vi "MakeBeverage.vi"(8 "Error In":errorcluster, 10 "Type":T1, 11 "reference in":refnum<class "BeverageFlyweightFactory.lvclass">) -> (0 "Error Out":errorcluster, 2 "Return(LabVIEW Class)":refnum<class "IBeverage.lvclass">, 3 "reference out":refnum<class "BeverageFlyweightFactory.lvclass">)   [LabVIEW 2020, in "BeverageFlyweightFactory.lvclass"]
uses:
  BeverageFlyweightFactory.lvclass
  BeverageType.ctl
  IBeverage_interface/IBeverage.lvclass
  BubbleMilkTea_class/BubbleMilkTea.lvclass
  C:/Projects/DesignPatterns/FlyweightPattern2/IBeverage_interface/IBeverage.lvclass
  FoamMilkTea_class/FoamMilkTea.lvclass
  OolingMilkTea_class/OolingMilkTea.lvclass
  CoconutMilkTea_class/CoconutMilkTea.lvclass
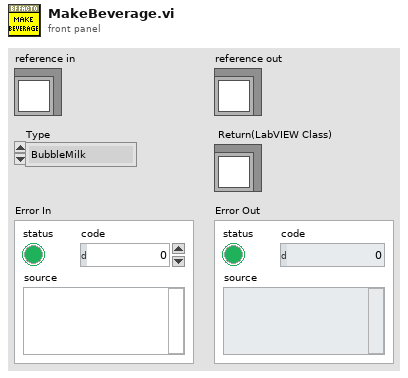
[diagram p1: front panel]
types:
  T1 = typedef "BeverageType.ctl" = enum16{"BubbleMilk", "FoamMilk", "OolongMilk", "CoconutMilk"}
  T2 = typedef "BeverageFlyweightFactory.lvclass/ObjectAttributes.ctl" = cluster{"_beverages":map{T1, refnum<class "IBeverage.lvclass">}}
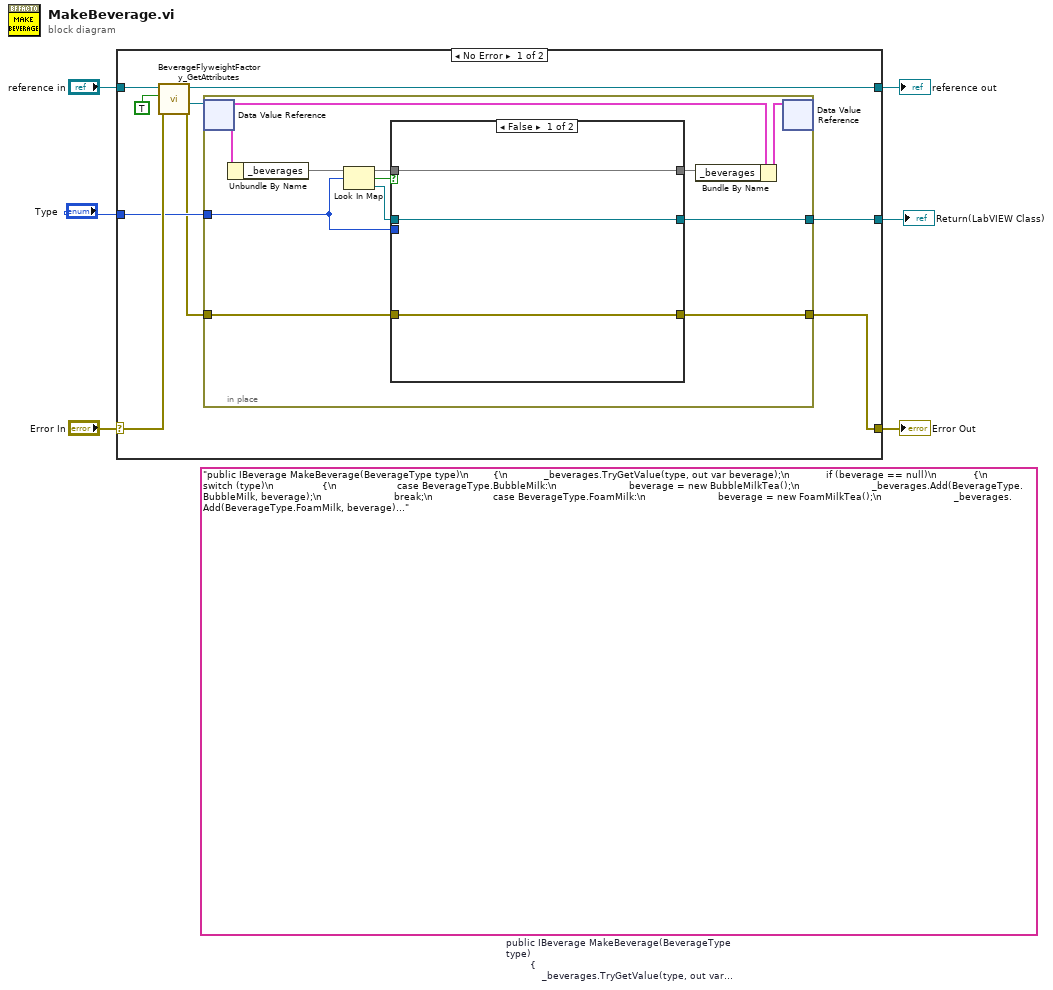
[diagram p0: block diagram]
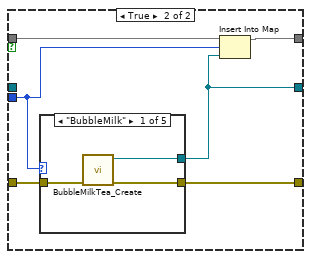
[diagram p2: hidden frame]
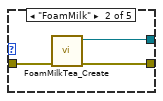
[diagram p3: hidden frame]
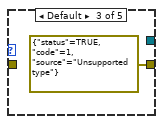
[diagram p4: hidden frame]
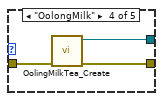
[diagram p5: hidden frame]
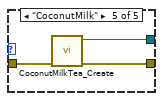
[diagram p6: hidden frame]
diagram:
  (unwired) "public IBeverage MakeBeverage(BeverageType type)\n        {\n            _beverages.TryGetValue(type, out var beverage);\n            if (beverage == null)\n            {\n                switch (type)\n                {\n                    case BeverageType.BubbleMilk:\n                        beverage = new BubbleMilkTea();\n                        _beverages.Add(BeverageType.BubbleMilk, beverage);\n                        break;\n                    case BeverageType.FoamMilk:\n                        beverage = new FoamMilkTea();\n                        _beverages.Add(BeverageType.FoamMilk, beverage);\n                        break;\n                    case BeverageType.OolongMilk:\n                        beverage = new OolingMilkTea();\n                        _beverages.Add(BeverageType.OolongMilk, beverage);\n                        break;\n                    case BeverageType.CoconutMilk:\n                        beverage = new CoconutMilkTea();\n                        _beverages.Add(BeverageType.CoconutMilk, beverage);\n                        break;\n                    default:\n                        throw new ArgumentOutOfRangeException(nameof(type), type, null);\n                }\n            }\n\n            return beverage;\n        }"  # public IBeverage MakeBeverage(BeverageType type)         {             _beverages.TryGetValue(type, out var beverage);             if (beverage == null)             {                 switch (type)                 {                     case BeverageType.BubbleMilk:                         beverage = new BubbleMilkTea();                         _beverages.Add(BeverageType.BubbleMilk, beverage);                         break;                     case BeverageType.FoamMilk:                         beverage = new FoamMilkTea();                         _beverages.Add(BeverageType.FoamMilk, beverage);                         break;                     case BeverageType.OolongMilk:                         beverage = new OolingMilkTea();                         _beverages.Add(BeverageType.OolongMilk, beverage);                         break;                     case BeverageType.CoconutMilk:                         beverage = new CoconutMilkTea();                         _beverages.Add(BeverageType.CoconutMilk, beverage);                         break;                     default:                         throw new ArgumentOutOfRangeException(nameof(type), type, null);                 }             }              return beverage;         }
  n1 = case shown="No Error" "Error In" {
    selector: "Error In" -> [w14 w49]
    tunnel: [w7 w49] -> w5
    tunnel: [w13 w48] -> w3
    tunnel: "reference in" -> [w15 w48]
    tunnel: "Type" -> [w10 _]
    tunnel: [w9 _] -> w1
    frame No Error {
      n2 = call "BeverageFlyweightFactory_GetAttributes.vi"("error in (no error)"=w14, "OnlyGetDvrReference(False)"=TRUE, "reference in"=w15) -> ("error out"=w8:errorcluster, "DataRef"=w12:refnum<data-value>, "reference out"=w13:refnum<class "BeverageFlyweightFactory.lvclass">)  [unwired: 5 in, 1 out]
      n3 = in-place {
        in-place-border: w10 -> [w18]
        in-place-border: [w19] -> w9
        in-place-border: w8 -> [w17]
        in-place-border: [w16] -> w7
        n4 = in-place-dvr #1(w12) -> (w24:T2)  [unwired: 1 out]
        n5 = Unbundle By Name(w24) -> ("_beverages"=w22:map{T1, refnum<class "IBeverage.lvclass">})
        n6 = Look In Map(map=w22, key=w18) -> (key not found?=w23:bool, value=w20:refnum<class "IBeverage.lvclass">)  [unwired: 1 in]
        n7 = case shown="False" w23 {
          tunnel: w22 -> [w28 w34]
          tunnel: [w28 w29] -> w21
          tunnel: [w27 w30] -> w19
          tunnel: w20 -> [w27 _]
          tunnel: w18 -> [_ w33]
          tunnel: w17 -> [w26 w32]
          tunnel: [w26 w31] -> w16
          frame False {
          }
          frame True {
            n8 = case shown="\"BubbleMilk\"" w33 {
              tunnel: [w37 w40 _ w44 w47] -> w30
              tunnel: w32 -> [w36 w39 _ w43 w46]
              tunnel: [w35 w38 errorcluster {"status"=TRUE, "code"=1, "source"="Unsupported type"} ("Error Out") w42 w45] -> w31
              frame "BubbleMilk" {
                n9 = call "BubbleMilkTea_Create.vi"("Error In"=w36) -> ("Error Out"=w35:errorcluster, "reference out"=w37:refnum<class "BubbleMilkTea.lvclass">)  [unwired: 9 in]
              }
              frame "FoamMilk" {
                n10 = call "FoamMilkTea_Create.vi"("Error In"=w39) -> ("Error Out"=w38:errorcluster, "reference out"=w40:refnum<class "FoamMilkTea.lvclass">)  [unwired: 9 in]
              }
              frame Default {
              }
              frame "OolongMilk" {
                n11 = call "OolingMilkTea_Create.vi"("Error In"=w43) -> ("Error Out"=w42:errorcluster, "reference out"=w44:refnum<class "OolingMilkTea.lvclass">)  [unwired: 9 in]
              }
              frame "CoconutMilk" {
                n12 = call "CoconutMilkTea_Create.vi"("Error In"=w46) -> ("Error Out"=w45:errorcluster, "reference out"=w47:refnum<class "CoconutMilkTea.lvclass">)  [unwired: 9 in]
              }
            }
            n13 = Insert Into Map(map in=w34, key=w33, value=w30) -> (map out=w29:map{T1, refnum<class "IBeverage.lvclass">})  [unwired: 2 out]
          }
        }
        n14 = Bundle By Name(cluster=w24, "_beverages"=w21) -> (w25:T2)
        n15 = in-place-dvr #1(w25) -> ()  [unwired: 2 out]
      }
    }
    frame Error {
    }
  }
  "Error Out" <- w5
  "reference out" <- w3
  "Return(LabVIEW Class)" <- w1
